vi "TankDrive.vi"(6 "HalfSpeed":bool=TRUE, 7 "Action":T1, 8 "Error In (no error)":errorcluster, 9 "Right Motor Value":dbl, 10 "Left Motor Value":dbl, 11 "RobotDriveDevRef":T2={"DevStatus"={"status"=FALSE, "code"=0, "source"=""}, "Motors[]"=[], "Square Inputs"=FALSE, "Max Output"=1.0, "Isochronous"=FALSE}) -> (0 "Error Out":errorcluster)   [LabVIEW 2012]
doc: "Sets tank drive inputs based on the given action. \nActions:\n-Init: sets the motor values to 0. This is the only time the motor reference is needed; it will be saved for future use.\n-SetValue: sets the motor values to the given values."
uses:
  <vilib>/Rock Robotics/WPI/RobotDrive/WPI_RobotDriveDevRef.ctl
  <vilib>/Rock Robotics/WPI/MotorControl/WPI_MotorControlDeviceRef.ctl
  <vilib>/Rock Robotics/SystemInterfaces/Typedef/FPGA_TypedefDigitalModule.ctl
  <vilib>/Rock Robotics/SystemInterfaces/DIO/FPGA_DIOPWMChannel.ctl
  <vilib>/Rock Robotics/WPI/PWM/WPI_PWMDeadband.ctl
  <vilib>/Rock Robotics/WPI/CAN/Jaguar/SubVIs/WPI_CANJaguar_ControlMode.ctl
  <vilib>/Rock Robotics/WPI/PWM/WPI_PWMTransform_ConPane.ctl
  ActionEnum.ctl
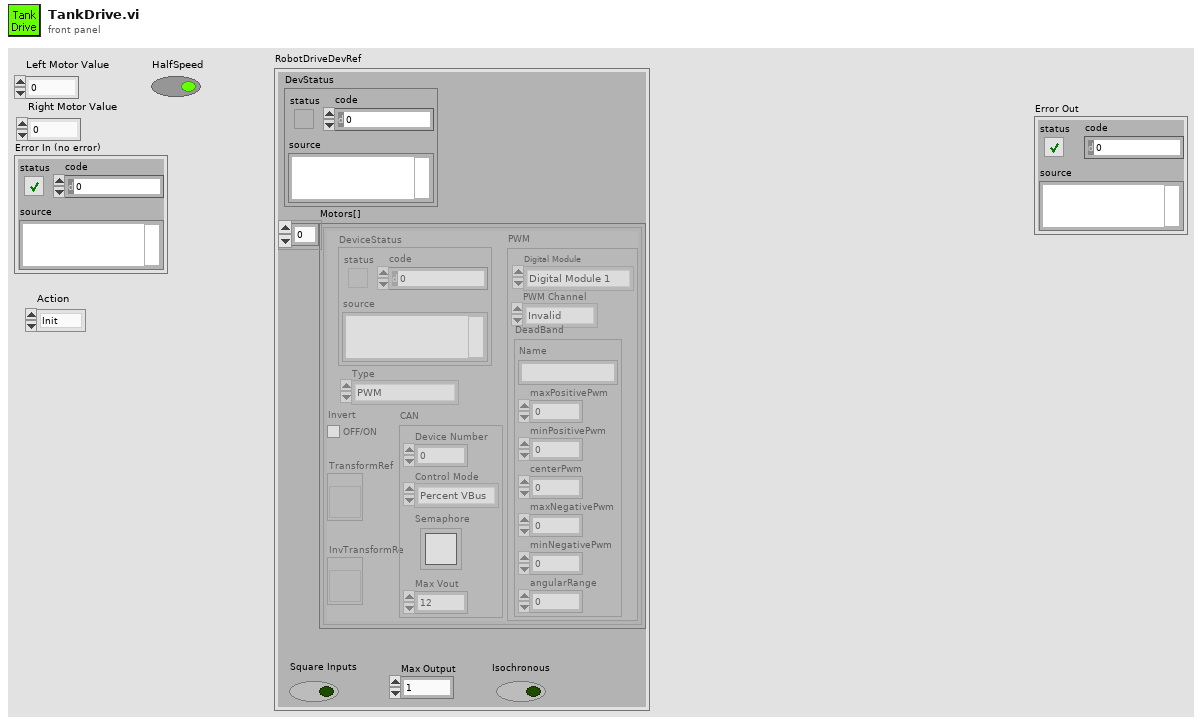
[diagram p1: front panel]
types:
  T1 = typedef "ActionEnum.ctl" = enum16{"Init", "SetValue"}
  T2 = typedef "WPI_RobotDriveDevRef.ctl" = cluster{"DevStatus":errorcluster, "Motors[]":T3[], "Square Inputs":bool, "Max Output":dbl, "Isochronous":bool}
  T3 = typedef "WPI_MotorControlDeviceRef.ctl" = cluster{"DeviceStatus":errorcluster, "Type":enum16{"PWM", "CAN"}, "PWM":cluster{"Digital Module":T4, "PWM Channel":T5, "DeadBand":T6}, "CAN":cluster{"Device Number":u8, "Control Mode":T7, "Semaphore":T8, "Max Vout":dbl}, "Invert":bool, "TransformRef":T9, "InvTransformRef":T9}
  T4 = typedef "FPGA_TypedefDigitalModule.ctl" = enum16{"Digital Module 1", "Digital Module 2"}
  T5 = typedef "FPGA_DIOPWMChannel.ctl" = enum8{"PWM 1", "PWM 2", "PWM 3", "PWM 4", "PWM 5", "PWM 6", "PWM 7", "PWM 8", "PWM 9", "PWM 10", "Invalid"}
  T6 = typedef "WPI_PWMDeadband.ctl" = cluster{"Name":string, "maxPositivePwm":i32, "minPositivePwm":i32, "centerPwm":i32, "maxNegativePwm":i32, "minNegativePwm":i32, "angularRange":u16}
  T7 = typedef "WPI_CANJaguar_ControlMode.ctl" = enum8{"Percent VBus", "Current", "Speed", "Position", "Voltage"}
  T8 = typedef "Semaphore RefNum" = refnum<k1>
  T9 = typedef "WPI_PWMTransform_ConPane.ctl" = refnum<vi>
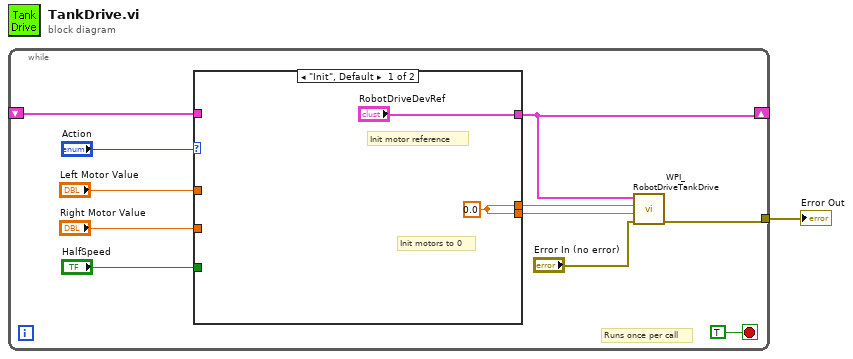
[diagram p0: block diagram]
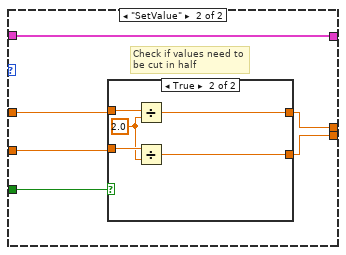
[diagram p2: hidden frame]
diagram:
  n1 = while {
    tunnel: [w11] -> w1
    shift-right: [w3] -> _
    shift-left: _ -> [w2]
    stop <- TRUE stop-if-true
    # "Runs once per call"
    n2 = case shown="\"Init\", Default" "Action" {
      tunnel: "HalfSpeed" -> [_ w20]
      tunnel: "Right Motor Value" -> [_ w19]
      tunnel: "Left Motor Value" -> [_ w18]
      tunnel: [w14 w17] -> w6
      tunnel: [w14 w16] -> w5
      tunnel: ["RobotDriveDevRef" w15] -> w3
      tunnel: w2 -> [_ w15]
      frame "Init", Default {
        w14 = 0.0
        # "Init motors to 0"
        # "Init motor reference"
      }
      frame "SetValue" {
        # "Check if values need to \nbe cut in half"
        n3 = case shown="True" w20 {
          tunnel: w19 -> [w22 w26]
          tunnel: w18 -> [w21 w27]
          tunnel: [w21 w24] -> w17
          tunnel: [w22 w23] -> w16
          frame False {
          }
          frame True {
            w25 = 2.0
            n4 = Divide(x=w27, y=w25) -> (x/y=w24:dbl)
            n5 = Divide(x=w26, y=w25) -> (x/y=w23:dbl)
          }
        }
      }
    }
    n6 = call <vilib>:"WPI_RobotDriveTankDrive.vi"("error in (no error)"="Error In (no error)", "Right axis value"=w5, "Left axis value"=w6, "RobotDriveDevRef"=w3) -> ("error out"=w11:errorcluster)  [unwired: 5 in, 2 out]
  }
  "Error Out" <- w1
